vi "XYMovingPartModifying_WangYunong.vi"() -> ()   [LabVIEW 2013]
uses:
  <vilib>/Instr/_visa.llb/VISA Configure Serial Port (Instr).vi
panel:
  out "concatenated string":string
  out "read buffer":string
  out "Array 2":dbl[](array[numeric])
  out "Time2":dbl
  out "x+y":dbl
  out "Array":dbl[][](array[numeric])
  in  "stop":bool
  out "Rod Pos?":cluster{dbl[], dbl[]}(graph)
  in  "X pole":refnum<visa-resource-name>
  in  "Y pole":refnum<visa-resource-name>
  in  "Mov speed(mm/s)":dbl format="%#_13g"
  out "y resolution":dbl
  out "x resolution":dbl
  out "XY Graph":cluster{dbl[], dbl[]}(graph)
  in  "Y Center / mm":dbl format="%#_13g"
  in  "X Center / mm":dbl format="%#_13g"
  in  "Size input solution":enum16{"Dynamic Size", "Fixed Size"}(ring)=enum."Fixed Size"
  out "Time":dbl
  in  "Shape":enum16{"Self-defined", "Circle"}(ring)=enum."Circle"
  in  "Radius / mm":dbl format="%#_13g"
  in  "Precision":i32
  in  "Polygon Point":dbl[][](array[numeric])
  out "X":i32
  out "Y":i32
  out "Case":i16
  out "x-y":u32
  in  "Y move Maximum / mm":dbl
  in  "X move Maximum / mm":dbl
  in  "Y step / mm":dbl
  in  "X step / mm":dbl
  in  "Initial YPos / mm":dbl
  in  "Initial XPos / mm":dbl
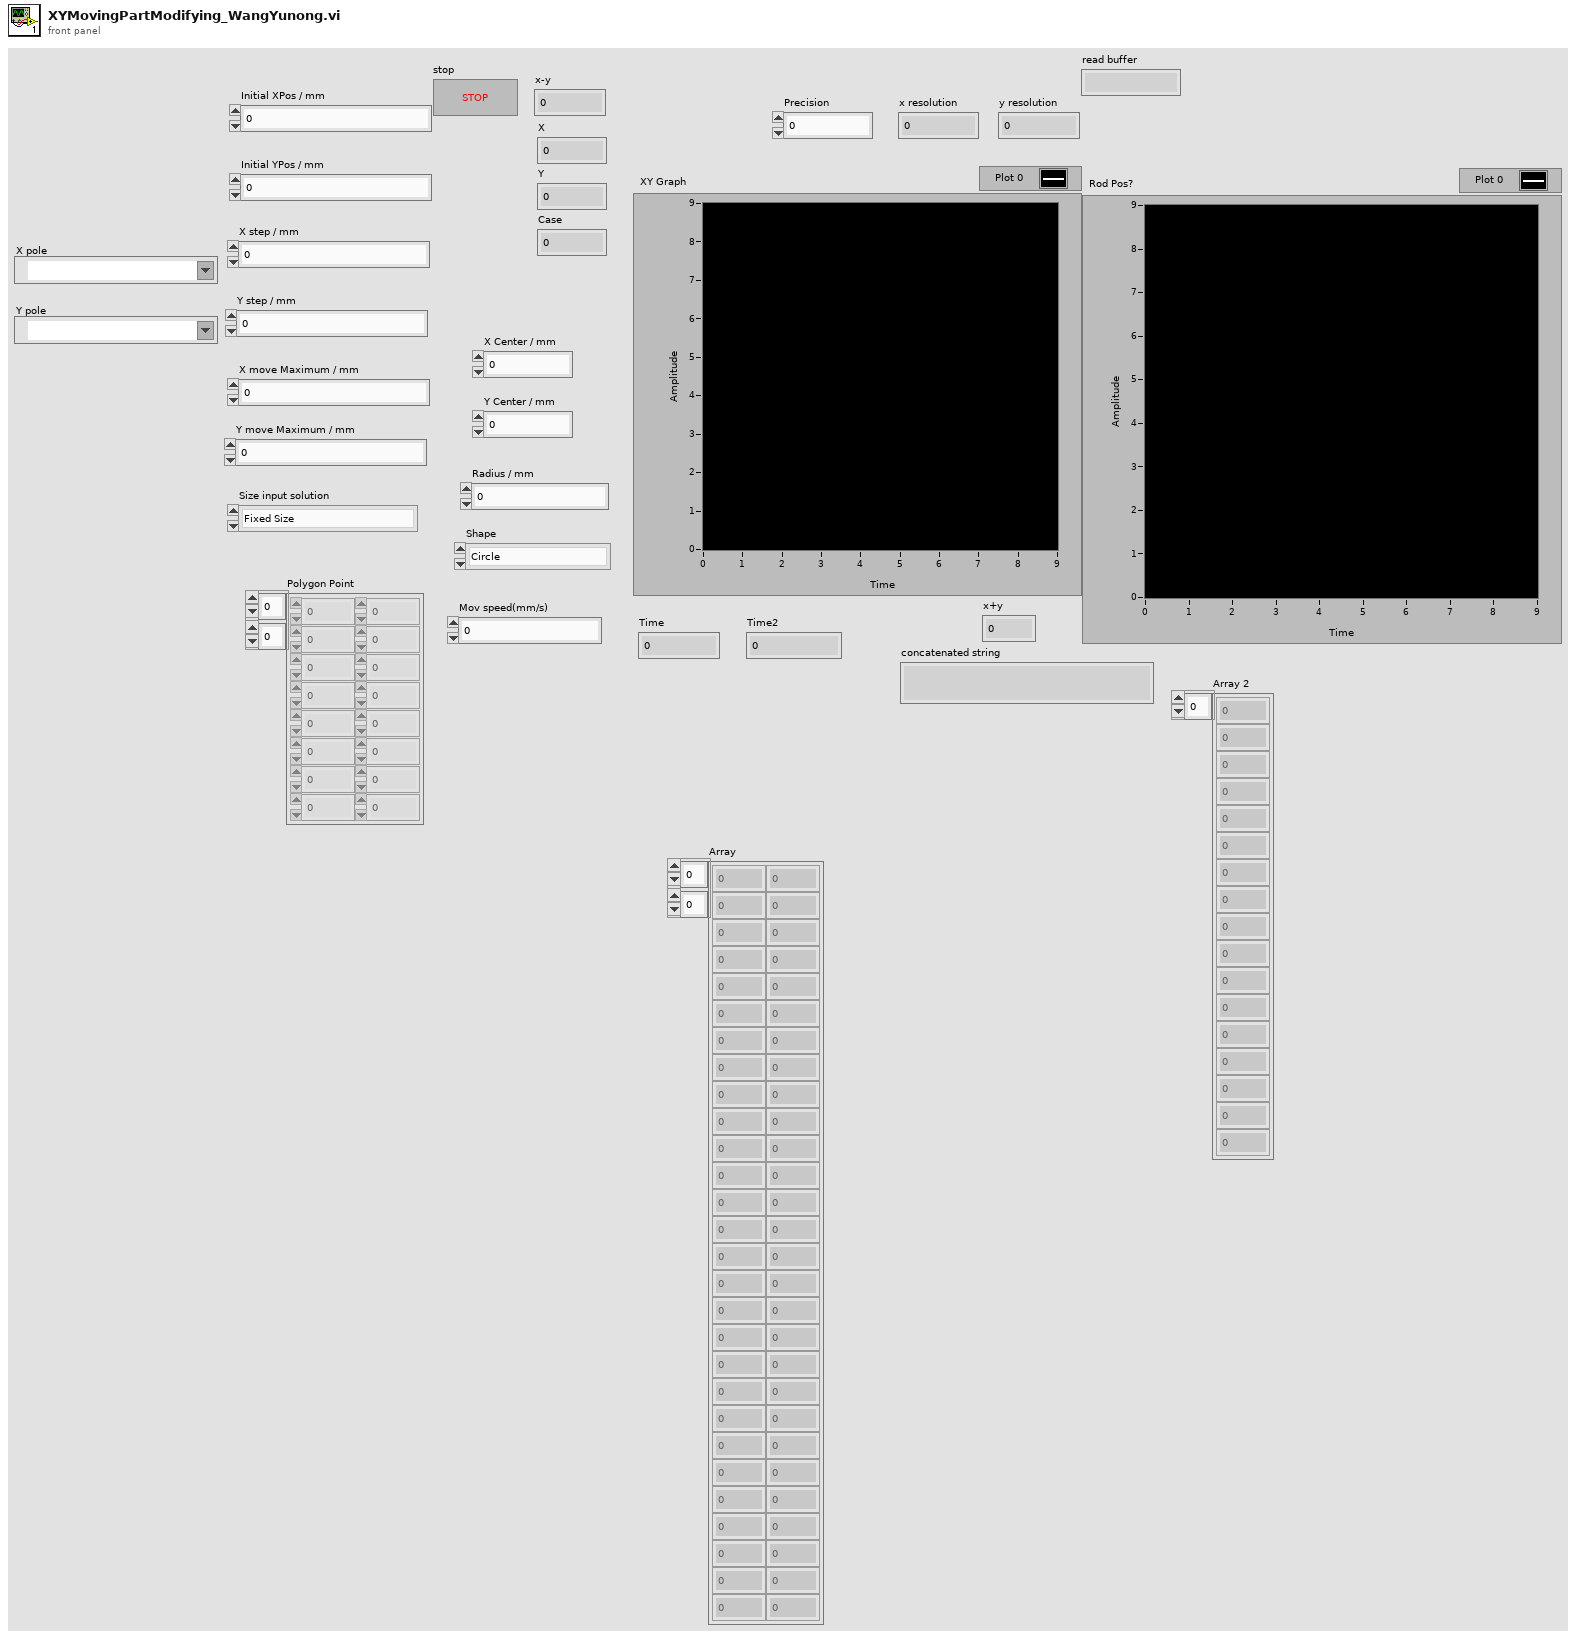
[diagram p1: front panel]
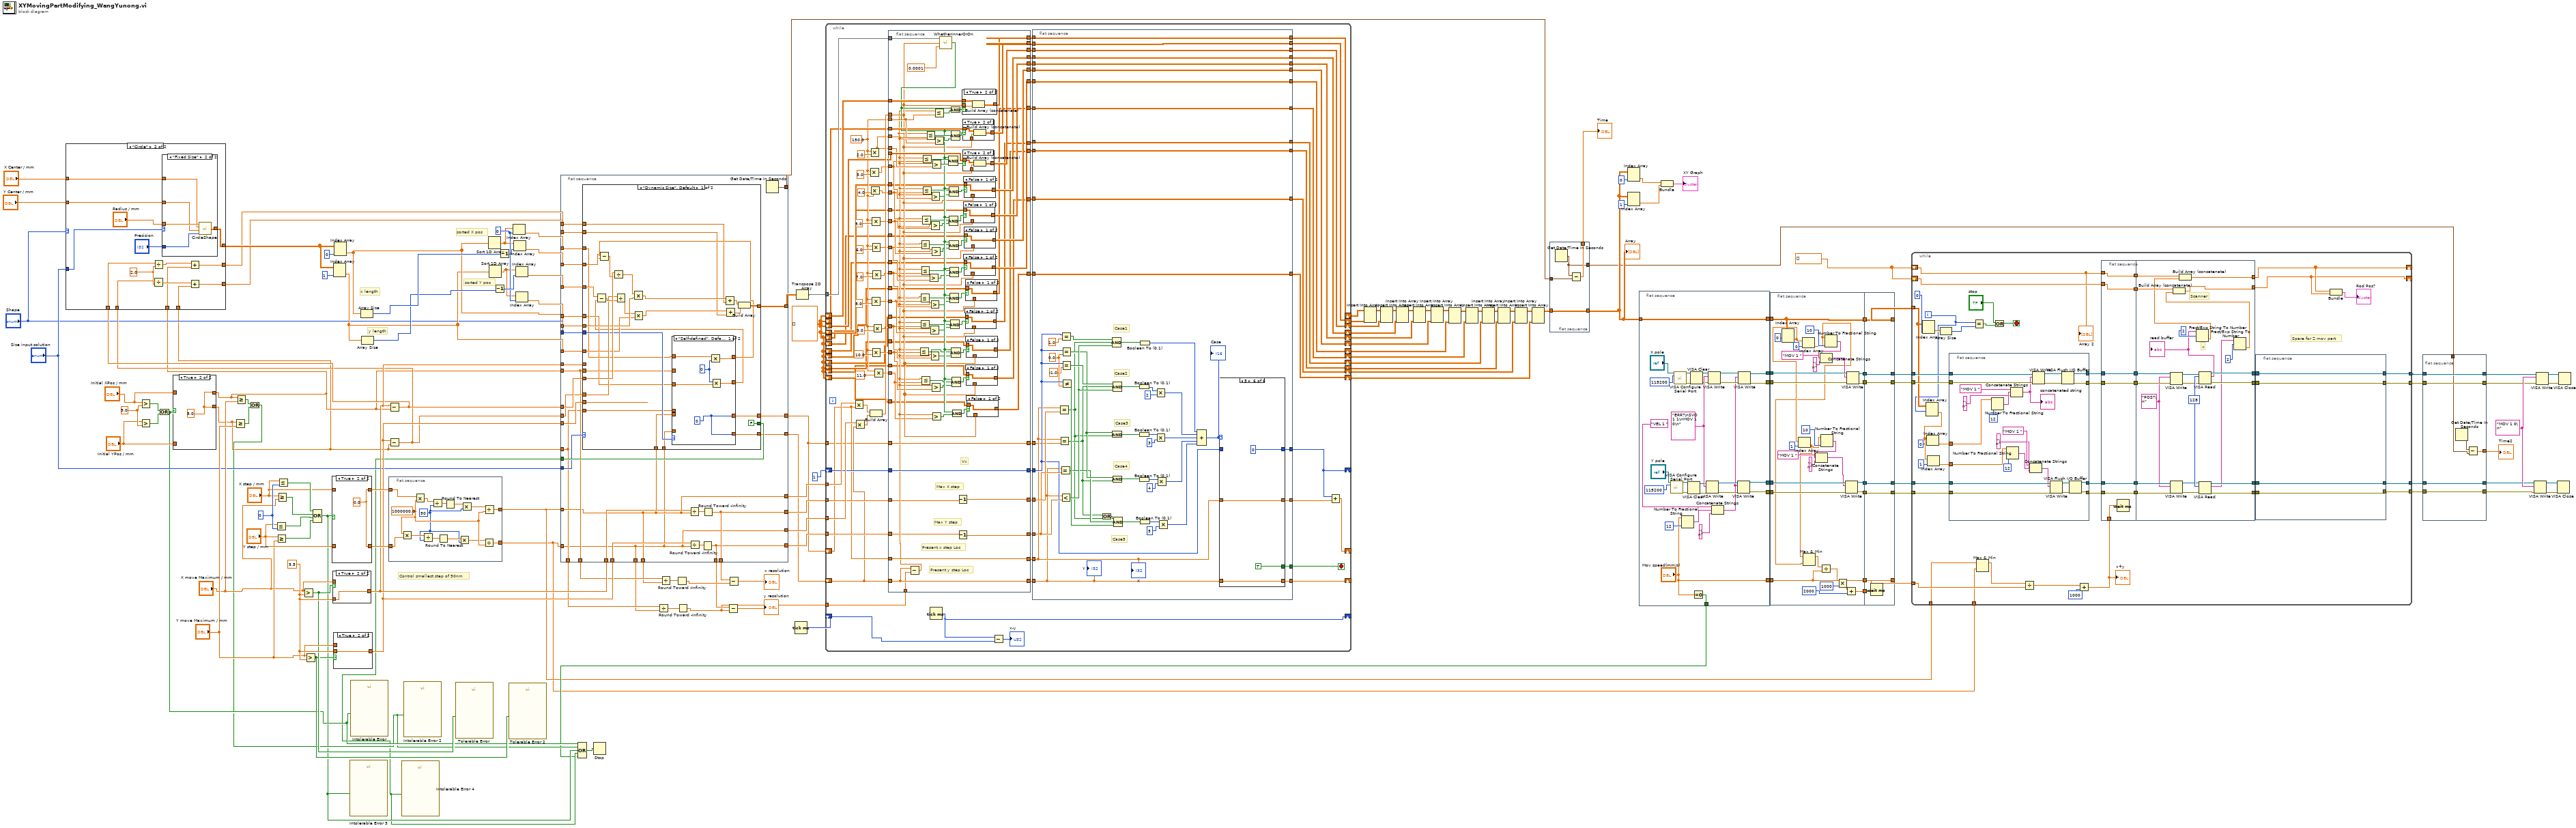
[diagram p0: block diagram]
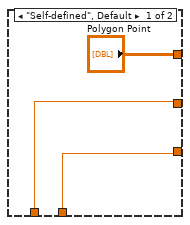
[diagram p2: hidden frame]
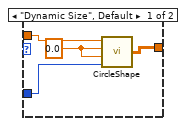
[diagram p3: hidden frame]
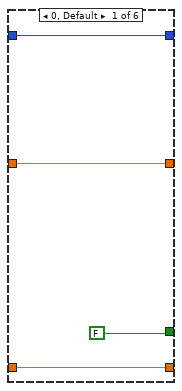
[diagram p4: hidden frame]
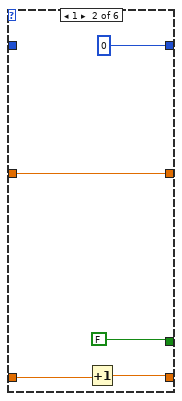
[diagram p5: hidden frame]
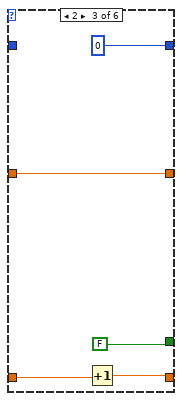
[diagram p6: hidden frame]
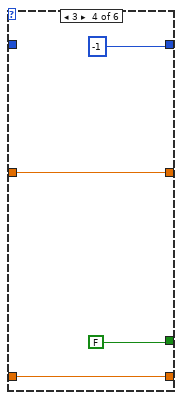
[diagram p7: hidden frame]
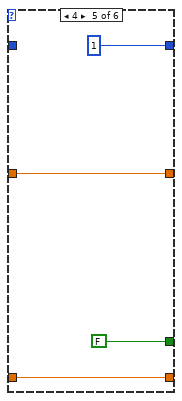
[diagram p8: hidden frame]
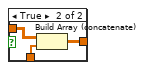
[diagram p9: hidden frame]
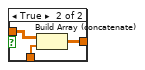
[diagram p10: hidden frame]
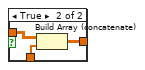
[diagram p11: hidden frame]
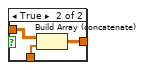
[diagram p12: hidden frame]
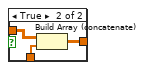
[diagram p13: hidden frame]
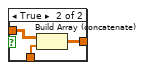
[diagram p14: hidden frame]
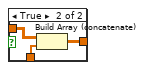
[diagram p15: hidden frame]
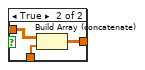
[diagram p16: hidden frame]
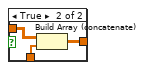
[diagram p17: hidden frame]
diagram:
  w26 = "MOV 1 0\n"
  w21 = dbl[] []
  w95 = 0 ("index")
  w61 = dbl[][] []
  w140 = 0
  w141 = 9.5
  w146 = 5.0
  # "sorted Y pos"
  # "sorted X pos"
  # "Control smallest step of 50nm"
  # "y length"
  # "x length"
  n1 = Greater?(x="Initial XPos / mm", y=w146) -> (0:w145:bool)
  n2 = Greater?(x="Initial YPos / mm", y=w146) -> (0:w144:bool)
  n3 = Or(x=w145, y=w144) -> (x .or. y?=w102:bool)
  n4 = case shown="True" w102 {
    tunnel: "Initial XPos / mm" -> [w148 _]
    tunnel: "Initial YPos / mm" -> [w147 _]
    tunnel: [w148 w149] -> w83
    tunnel: [w147 w149] -> w82
    frame False {
    }
    frame True {
      w149 = 5.0
    }
  }
  n5 = Greater Or Equal?(x=w82, y="Y move Maximum / mm") -> (x >= y?=w128:bool)
  n6 = Greater Or Equal?(x=w83, y="X move Maximum / mm") -> (x >= y?=w129:bool)
  n7 = Or(x=w129, y=w128) -> (x .or. y?=w101:bool)
  n8 = Less Or Equal?(x="Y step / mm", y=w140) -> (x <= y?=w137:bool)
  n9 = Greater Or Equal?(x="Y step / mm", y="Y move Maximum / mm") -> (x >= y?=w136:bool)
  n10 = Greater Or Equal?(x="X step / mm", y="X move Maximum / mm") -> (x >= y?=w138:bool)
  n11 = Less Or Equal?(x="X step / mm", y=w140) -> (x <= y?=w139:bool)
  n12 = Greater?(x="X move Maximum / mm", y=w141) -> (0:w127:bool)
  n13 = Greater?(x="Y move Maximum / mm", y=w141) -> (0:w126:bool)
  n14 = Compound Arithmetic op=OR(w139, w138, w137, w136) -> (w100:bool)
  n15 = case shown="True" w100 {
    tunnel: "X step / mm" -> [w151 _]
    tunnel: "Y step / mm" -> [w150 _]
    tunnel: [w151 w152] -> w125
    tunnel: [w150 w152] -> w124
    frame False {
    }
    frame True {
      w152 = 0.0
    }
  }
  n16 = case shown="True" w127 {
    tunnel: w141 -> [_ w154]
    tunnel: "X move Maximum / mm" -> [w153 _]
    tunnel: [w153 w154] -> w115
    frame False {
    }
    frame True {
    }
  }
  n17 = case shown="True" w126 {
    tunnel: w141 -> [_ w156]
    tunnel: "Y move Maximum / mm" -> [w155 _]
    tunnel: [w155 w156] -> w114
    frame False {
    }
    frame True {
    }
  }
  n18 = call "Intolerable Error 3"("Enable"=w100) -> ()  [unwired: 9 in, 2 out]
  n19 = call "Intolerable Error"("Enable"=w102) -> ()  [unwired: 9 in, 2 out]
  n20 = Subtract(x=w115, y=w83) -> (x-y=w108:dbl)
  n21 = Subtract(x=w114, y=w82) -> (x-y=w107:dbl)
  n22 = case shown="\"Circle\"" "Shape" {
    tunnel: ["Polygon Point" w172] -> w117
    tunnel: "Size input solution" -> [_ w171]
    tunnel: w108 -> [_ w167]
    tunnel: w107 -> [_ w166]
    tunnel: w82 -> [w157 w165]
    tunnel: w83 -> [w158 w164]
    tunnel: [w158 w163] -> w106
    tunnel: [w157 w162] -> w105
    tunnel: "X Center / mm" -> [_ w161]
    tunnel: "Y Center / mm" -> [_ w160]
    frame "Self-defined", Default {
    }
    frame "Circle" {
      w170 = 2.0
      n23 = Divide(x=w166, y=w170) -> (x/y=w168:dbl)
      n24 = Divide(x=w167, y=w170) -> (x/y=w169:dbl)
      n25 = case shown="\"Fixed Size\"" w171 {
        tunnel: "Radius / mm" -> [w177 w183]
        tunnel: "Precision" -> [w176 w182]
        tunnel: [w178 w181] -> w172
        tunnel: w161 -> [_ w180]
        tunnel: w160 -> [_ w179]
        frame "Dynamic Size", Default {
          w175 = 0.0 ("X initial")
          n26 = call "CircleShape.vi"("Precision"=w176, "Y initial"=w175, "X initial"=w175, "Radius"=w177) -> ("Output Point"=w178:dbl[][])
        }
        frame "Fixed Size" {
          n27 = call "CircleShape.vi"("Precision"=w182, "Y initial"=w179, "X initial"=w180, "Radius"=w183) -> ("Output Point"=w181:dbl[][])
        }
      }
      n28 = Add(x=w169, y=w164) -> (x+y=w163:dbl)
      n29 = Add(x=w168, y=w165) -> (x+y=w162:dbl)
    }
  }
  n30 = Index Array(array=w117, index (col)=1 ("disabled index (col)")) -> (element=w85:dbl[])  [unwired: 1 in]
  n31 = Index Array(array=w117, index (col)=0 ("disabled index (col)")) -> (element=w86:dbl[])  [unwired: 1 in]
  n32 = Array Size(array=w86) -> (size(s)=w88:i32)
  n33 = Array Size(array=w85) -> (size(s)=w87:i32)
  n34 = flat-sequence {
    tunnel: w125 -> [w197]
    tunnel: w124 -> [w194]
    tunnel: [w190] -> w20
    tunnel: [w189] -> w19
    frame #0 {
      w186 = 50
      w191 = 1000000.0
      n35 = Multiply(x=w191, y=w194) -> (x*y=w193:dbl)
      n36 = Multiply(x=w197, y=w191) -> (x*y=w196:dbl)
      n37 = Divide(x=w193, y=w186) -> (x/y=w192:dbl)
      n38 = Divide(x=w196, y=w186) -> (x/y=w195:dbl)
      n39 = Round To Nearest(number=w192) -> (nearest integer value=w187:dbl)
      n40 = Round To Nearest(number=w195) -> (nearest integer value=w188:dbl)
      n41 = Multiply(x=w187, y=w186) -> (x*y=w185:dbl)
      n42 = Multiply(x=w188, y=w186) -> (x*y=w184:dbl)
      n43 = Divide(x=w185, y=w191) -> (x/y=w189:dbl)
      n44 = Divide(x=w184, y=w191) -> (x/y=w190:dbl)
    }
  }
  n45 = call "Intolerable Error 4"("Enable"=w99) -> ()  [unwired: 9 in, 2 out]
  n46 = call "Intolerable Error 2"("Enable"=w101) -> ()  [unwired: 9 in, 2 out]
  n47 = call "Tolerable Error"("Enable"=w127) -> ()  [unwired: 9 in, 2 out]
  n48 = Sort 1D Array(array=w86) -> (sorted array=w93:dbl[])
  n49 = Sort 1D Array(array=w85) -> (sorted array=w94:dbl[])
  n50 = Decrement(x=w87) -> (x-1=w96:i32)
  n51 = Decrement(x=w88) -> (x-1=w97:i32)
  n52 = call "Tolerable Error 2"("Enable"=w126) -> ()  [unwired: 9 in, 2 out]
  n53 = Index Array(array=w93, index=w95) -> (element=w92:dbl)
  n54 = Index Array(array=w93, index=w97) -> (element=w91:dbl)
  n55 = Index Array(array=w94, index=w96) -> (element=w90:dbl)
  n56 = Index Array(array=w94, index=w95) -> (element=w89:dbl)
  n57 = flat-sequence {
    tunnel: w108 -> [w220]
    tunnel: w107 -> [w219]
    tunnel: w115 -> [w226]
    tunnel: w83 -> [w203]
    tunnel: w114 -> [w225]
    tunnel: w82 -> [w199]
    tunnel: [w224] -> w99
    tunnel: w20 -> [w202]
    tunnel: w19 -> [w198]
    tunnel: [w223] -> w119
    tunnel: [w201] -> w123
    tunnel: [w200] -> w122
    tunnel: [w198] -> w121
    tunnel: [w202] -> w120
    tunnel: [w218] -> w116
    tunnel: w106 -> [w217]
    tunnel: w105 -> [w216]
    tunnel: w115 -> [w215]
    tunnel: w114 -> [w214]
    tunnel: [w213] -> w110
    tunnel: [w212] -> w111
    tunnel: "Size input solution" -> [w211]
    tunnel: w92 -> [w210]
    tunnel: w91 -> [w209]
    tunnel: w90 -> [w208]
    tunnel: w89 -> [w207]
    tunnel: w86 -> [w206]
    tunnel: w85 -> [w205]
    tunnel: "Shape" -> [w204]
    tunnel: [w203] -> w72
    tunnel: [w202] -> w71
    tunnel: [w201] -> w69
    tunnel: [w200] -> w65
    tunnel: [w199] -> w64
    tunnel: [w198] -> w63
    frame #0 {
      n58 = case shown="\"Dynamic Size\", Default" w211 {
        tunnel: w206 -> [w249 w277]
        tunnel: w205 -> [w248 w276]
        tunnel: w209 -> [w255 w292]
        tunnel: w210 -> [w234 w290]
        tunnel: w208 -> [w254 w288]
        tunnel: w207 -> [w232 w285]
        tunnel: w220 -> [w253 _]
        tunnel: w219 -> [w250 _]
        tunnel: [w235 w278] -> w223
        tunnel: w226 -> [_ w291]
        tunnel: w203 -> [w243 w289]
        tunnel: w225 -> [_ w287]
        tunnel: w199 -> [w242 w286]
        tunnel: [FALSE w279] -> w224
        tunnel: w217 -> [w227 _]
        tunnel: w216 -> [w228 _]
        tunnel: w202 -> [w241 _]
        tunnel: w198 -> [w240 _]
        tunnel: [w238 w275] -> w213
        tunnel: [w239 w275] -> w212
        tunnel: w204 -> [w244 _]
        frame "Dynamic Size", Default {
          n59 = case shown="\"Self-defined\", Default" w244 {
            tunnel: w243 -> [_ w272]
            tunnel: w242 -> [_ w271]
            tunnel: w241 -> [_ w270]
            tunnel: w240 -> [_ w269]
            tunnel: [w261 w268] -> w239
            tunnel: [w261 w267] -> w238
            tunnel: w234 -> [w260 w266]
            tunnel: [w257 w265] -> w233
            tunnel: w232 -> [w259 w264]
            tunnel: [w256 w262] -> w231
            frame "Self-defined", Default {
              w258 = 0
              w261 = 0
              n60 = Multiply(x=w260, y=w258) -> (x*y=w257:dbl)
              n61 = Multiply(x=w258, y=w259) -> (x*y=w256:dbl)
            }
            frame "Circle" {
              w263 = 1.0
              n62 = Divide(x=w271, y=w269) -> (x/y=w273:dbl)
              n63 = Divide(x=w272, y=w270) -> (x/y=w274:dbl)
              n64 = Multiply(x=w266, y=w263) -> (x*y=w265:dbl)
              n65 = Multiply(x=w263, y=w264) -> (x*y=w262:dbl)
              n66 = Round Toward -Infinity(1:w274) -> (0:w268:dbl)
              n67 = Round Toward -Infinity(1:w273) -> (0:w267:dbl)
            }
          }
          n68 = Subtract(x=w254, y=w231) -> (x-y=w251:dbl)
          n69 = Subtract(x=w255, y=w233) -> (x-y=w252:dbl)
          n70 = Divide(x=w253, y=w252) -> (x/y=w230:dbl)
          n71 = Divide(x=w250, y=w251) -> (x/y=w229:dbl)
          n72 = Multiply(x=w230, y=w249) -> (x*y=w246:dbl[])
          n73 = Multiply(x=w229, y=w248) -> (x*y=w245:dbl[])
          n74 = Add(x=w246, y=w227) -> (x+y=w237:dbl[])
          n75 = Add(x=w245, y=w228) -> (x+y=w236:dbl[])
          n76 = Build Array(w237, w236) -> (w235:dbl[][])
        }
        frame "Fixed Size" {
          w275 = 0
          n77 = Greater?(x=w292, y=w291) -> (0:w283:bool)
          n78 = Less?(x=w290, y=w289) -> (x < y?=w284:bool)
          n79 = Greater?(x=w288, y=w287) -> (0:w282:bool)
          n80 = Less?(x=w285, y=w286) -> (x < y?=w281:bool)
          n81 = Compound Arithmetic op=OR(w284, w283, w282, w281) -> (w280:bool)
          n82 = case shown="True" w280 {
            tunnel: [FALSE TRUE] -> w279
            frame False {
            }
            frame True {
            }
          }
          n83 = Build Array(w277, w276) -> (w278:dbl[][])
        }
      }
      n84 = Divide(x=w215, y=w202) -> (x/y=w222:dbl)
      n85 = Divide(x=w214, y=w198) -> (x/y=w221:dbl)
      n86 = Round Toward -Infinity(1:w221) -> (0:w200:dbl)
      n87 = Round Toward -Infinity(1:w222) -> (0:w201:dbl)
      n88 = Get Date/Time In Seconds() -> (seconds since 1Jan1904=w218:timestamp)
    }
  }
  n89 = Compound Arithmetic op=OR(w102, w101, w100, w99, w27) -> (w98:bool)
  n90 = Stop(stop? (T)=w98) -> ()
  n91 = Divide(x=w64, y=w63) -> (x/y=w66:dbl)
  n92 = Divide(x=w72, y=w71) -> (x/y=w73:dbl)
  n93 = Round Toward -Infinity(1:w73) -> (0:w68:dbl)
  n94 = Round Toward -Infinity(1:w66) -> (0:w62:dbl)
  n95 = Subtract(x=w65, y=w62) -> (x-y=→"y resolution":dbl)
  n96 = Subtract(x=w69, y=w68) -> (x-y=→"x resolution":dbl)
  n97 = Tick Count (ms)() -> (millisecond timer value=w81:u32)
  n98 = Transpose 2D Array(2D array=w119) -> (transposed array=w118:dbl[][])
  n99 = while {
    tunnel: w123 -> [w367]
    tunnel: w122 -> [w365]
    tunnel: w118 -> [w373]
    tunnel: w121 -> [w377]
    tunnel: w120 -> [w378]
    shift-right: [w358] -> _
    shift-left: 1 -> [w369]
    shift-right: [w357] -> _
    shift-left: w111 -> [w363]
    shift-right: [w356] -> _
    shift-left: w110 -> [w361]
    shift-right: [w355] -> w75
    shift-left: w61 -> [w372]
    tunnel: w111 -> [w353]
    shift-right: [w351] -> _
    shift-left: w81 -> [w352]
    shift-right: [w347] -> w74
    shift-left: w61 -> [w346]
    tunnel: w62 -> [w345]
    shift-right: [w340] -> w55
    shift-left: w61 -> [w342]
    shift-right: [w319] -> w54
    shift-left: w61 -> [w321]
    shift-right: [w316] -> w53
    shift-left: w61 -> [w318]
    shift-right: [w313] -> w52
    shift-left: w61 -> [w315]
    shift-right: [w310] -> w51
    shift-left: w61 -> [w312]
    shift-right: [w307] -> w49
    shift-left: w61 -> [w309]
    shift-right: [w304] -> w47
    shift-left: w61 -> [w306]
    shift-right: [w301] -> w46
    shift-left: w61 -> [w303]
    shift-right: [w298] -> w44
    shift-left: w61 -> [w300]
    shift-right: [w295] -> w41
    shift-left: w61 -> [w297]
    stop <- w360 stop-if-true
    w329 = 150.0
    n100 = Multiply(x=w378, y=w363) -> (x*y=w376:dbl)
    n101 = Multiply(x=w377, y=w361) -> (x*y=w375:dbl)
    n102 = Multiply(x=w329, y=3.0) -> (x*y=w339:dbl)
    n103 = Multiply(x=w329, y=2.0) -> (x*y=w344:dbl)
    n104 = Multiply(x=w329, y=4.0) -> (x*y=w335:dbl)
    n105 = Multiply(x=w329, y=5.0) -> (x*y=w328:dbl)
    n106 = Multiply(x=w329, y=8.0) -> (x*y=w325:dbl)
    n107 = Multiply(x=w329, y=6.0) -> (x*y=w327:dbl)
    n108 = Multiply(x=w329, y=10.0) -> (x*y=w323:dbl)
    n109 = Build Array(w376, w375) -> (w374:dbl[])
    n110 = Multiply(x=w329, y=7.0) -> (x*y=w326:dbl)
    n111 = Multiply(x=w329, y=9.0) -> (x*y=w324:dbl)
    n112 = Multiply(x=w329, y=11.0) -> (x*y=w322:dbl)
    n113 = flat-sequence {
      tunnel: w374 -> [w491]
      tunnel: w373 -> [w538]
      tunnel: w372 -> [w528]
      tunnel: [w541] -> w371
      tunnel: [w540] -> w370
      tunnel: w369 -> [w540]
      tunnel: [w460] -> w368
      tunnel: w367 -> [w461]
      tunnel: [w458] -> w366
      tunnel: w365 -> [w459]
      tunnel: [w539] -> w364
      tunnel: w363 -> [w539]
      tunnel: [w525] -> w362
      tunnel: w361 -> [w525]
      tunnel: [w536] -> w354
      tunnel: w353 -> [w536]
      tunnel: w329 -> [w529]
      tunnel: w344 -> [w530]
      tunnel: [w527] -> w348
      tunnel: w346 -> [w526]
      tunnel: w345 -> [w524]
      tunnel: w344 -> [w518]
      tunnel: w342 -> [w520]
      tunnel: [w519] -> w341
      tunnel: w339 -> [w490]
      tunnel: w335 -> [w488]
      tunnel: w328 -> [w487]
      tunnel: w327 -> [w486]
      tunnel: w326 -> [w485]
      tunnel: w325 -> [w484]
      tunnel: w324 -> [w483]
      tunnel: w323 -> [w482]
      tunnel: w322 -> [w480]
      tunnel: w321 -> [w479]
      tunnel: [w478] -> w320
      tunnel: w318 -> [w477]
      tunnel: [w476] -> w317
      tunnel: w315 -> [w475]
      tunnel: [w474] -> w314
      tunnel: w312 -> [w473]
      tunnel: [w472] -> w311
      tunnel: w309 -> [w471]
      tunnel: [w470] -> w308
      tunnel: w306 -> [w469]
      tunnel: [w468] -> w305
      tunnel: w303 -> [w467]
      tunnel: [w466] -> w302
      tunnel: w300 -> [w465]
      tunnel: [w464] -> w299
      tunnel: w297 -> [w463]
      tunnel: [w462] -> w296
      frame #0 {
        # "Max X step"
        # "Max Y step"
        # "Present y step Loc"
        # "Present x step Loc"
        # "Vx"
        n114 = Subtract(x=w525, y=w524) -> (x-y=w481:dbl)
        n115 = Less Or Equal?(x=w481, y=w482) -> (x <= y?=w495:bool)
        n116 = Less Or Equal?(x=w481, y=w484) -> (x <= y?=w499:bool)
        n117 = Less Or Equal?(x=w481, y=w483) -> (x <= y?=w497:bool)
        n118 = Less Or Equal?(x=w481, y=w486) -> (x <= y?=w503:bool)
        n119 = Less Or Equal?(x=w481, y=w485) -> (x <= y?=w501:bool)
        n120 = Less Or Equal?(x=w481, y=w480) -> (x <= y?=w493:bool)
        n121 = Less Or Equal?(x=w481, y=w487) -> (x <= y?=w505:bool)
        n122 = Less Or Equal?(x=w481, y=w490) -> (x <= y?=w522:bool)
        n123 = Less Or Equal?(x=w481, y=w488) -> (x <= y?=w507:bool)
        n124 = Less Or Equal?(x=w481, y=w530) -> (x <= y?=w532:bool)
        n125 = Greater?(x=w481, y=w486) -> (0:w500:bool)
        n126 = Greater?(x=w481, y=w484) -> (0:w496:bool)
        n127 = Greater?(x=w481, y=w485) -> (0:w498:bool)
        n128 = Greater?(x=w481, y=w483) -> (0:w494:bool)
        n129 = Greater?(x=w481, y=w488) -> (0:w504:bool)
        n130 = Greater?(x=w481, y=w490) -> (0:w506:bool)
        n131 = Greater?(x=w481, y=w487) -> (0:w502:bool)
        n132 = Greater?(x=w481, y=w482) -> (0:w492:bool)
        n133 = Greater?(x=w481, y=w518) -> (0:w521:bool)
        n134 = Greater?(x=w481, y=w480) -> (0:w489:bool)
        n135 = Less Or Equal?(x=w481, y=w529) -> (x <= y?=w534:bool)
        n136 = Greater?(x=w481, y=w529) -> (0:w531:bool)
        n137 = call "WhetherInnerOrOn.vi"("Error permitted"=0.0001, "JudgePoint"=w491, "InputPolygon"=w538) -> ("Point on or inside?"=w508:bool)
        n138 = Compound Arithmetic op=AND(w508, w522, w521) -> (w523:bool)
        n139 = Compound Arithmetic op=AND(w508, w505, w504) -> (w516:bool)
        n140 = And(x=w508, y=w534) -> (x .and. y?=w535:bool)
        n141 = Compound Arithmetic op=AND(w508, w507, w506) -> (w517:bool)
        n142 = Compound Arithmetic op=AND(w508, w503, w502) -> (w515:bool)
        n143 = Compound Arithmetic op=AND(w508, w501, w500) -> (w514:bool)
        n144 = Compound Arithmetic op=AND(w508, w499, w498) -> (w513:bool)
        n145 = Compound Arithmetic op=AND(w508, w497, w496) -> (w512:bool)
        n146 = Compound Arithmetic op=AND(w508, w532, w531) -> (w533:bool)
        n147 = Compound Arithmetic op=AND(w508, w495, w494) -> (w511:bool)
        n148 = Compound Arithmetic op=AND(w508, w493, w492) -> (w510:bool)
        n149 = Compound Arithmetic op=AND(w508, w489) -> (w509:bool)
        n150 = Decrement(x=w461) -> (x-1=w460:dbl)
        n151 = Decrement(x=w459) -> (x-1=w458:dbl)
        n152 = case shown="True" w535 {
          tunnel: w528 -> [w586 w589]
          tunnel: w491 -> [_ w588]
          tunnel: [w586 w587] -> w541
          frame False {
          }
          frame True {
            n153 = Build Array (concatenate)(w589, w588) -> (w587:dbl[][])
          }
        }
        n154 = case shown="True" w533 {
          tunnel: w491 -> [_ w585]
          tunnel: w526 -> [w582 w584]
          tunnel: [w582 w583] -> w527
          frame False {
          }
          frame True {
            n155 = Build Array (concatenate)(w584, w585) -> (w583:dbl[][])
          }
        }
        n156 = case shown="True" w523 {
          tunnel: w491 -> [_ w581]
          tunnel: w520 -> [w578 w580]
          tunnel: [w578 w579] -> w519
          frame False {
          }
          frame True {
            n157 = Build Array (concatenate)(w580, w581) -> (w579:dbl[][])
          }
        }
        n158 = case shown="False" w516 {
          tunnel: w491 -> [_ w545]
          tunnel: [w542 w544] -> w476
          tunnel: w477 -> [w542 w543]
          frame False {
          }
          frame True {
            n159 = Build Array (concatenate)(w543, w545) -> (w544:dbl[][])
          }
        }
        n160 = case shown="False" w517 {
          tunnel: w491 -> [_ w577]
          tunnel: [w574 w576] -> w478
          tunnel: w479 -> [w574 w575]
          frame False {
          }
          frame True {
            n161 = Build Array (concatenate)(w575, w577) -> (w576:dbl[][])
          }
        }
        n162 = case shown="False" w514 {
          tunnel: w491 -> [_ w569]
          tunnel: [w566 w568] -> w472
          tunnel: w473 -> [w566 w567]
          frame False {
          }
          frame True {
            n163 = Build Array (concatenate)(w567, w569) -> (w568:dbl[][])
          }
        }
        n164 = case shown="False" w515 {
          tunnel: w491 -> [_ w573]
          tunnel: [w570 w572] -> w474
          tunnel: w475 -> [w570 w571]
          frame False {
          }
          frame True {
            n165 = Build Array (concatenate)(w571, w573) -> (w572:dbl[][])
          }
        }
        n166 = case shown="False" w512 {
          tunnel: w491 -> [_ w561]
          tunnel: [w558 w560] -> w468
          tunnel: w469 -> [w558 w559]
          frame False {
          }
          frame True {
            n167 = Build Array (concatenate)(w559, w561) -> (w560:dbl[][])
          }
        }
        n168 = case shown="False" w513 {
          tunnel: w491 -> [_ w565]
          tunnel: [w562 w564] -> w470
          tunnel: w471 -> [w562 w563]
          frame False {
          }
          frame True {
            n169 = Build Array (concatenate)(w563, w565) -> (w564:dbl[][])
          }
        }
        n170 = case shown="False" w511 {
          tunnel: w491 -> [_ w557]
          tunnel: [w554 w556] -> w466
          tunnel: w467 -> [w554 w555]
          frame False {
          }
          frame True {
            n171 = Build Array (concatenate)(w555, w557) -> (w556:dbl[][])
          }
        }
        n172 = case shown="False" w510 {
          tunnel: w491 -> [_ w553]
          tunnel: [w550 w552] -> w464
          tunnel: w465 -> [w550 w551]
          frame False {
          }
          frame True {
            n173 = Build Array (concatenate)(w551, w553) -> (w552:dbl[][])
          }
        }
        n174 = case shown="False" w509 {
          tunnel: w491 -> [_ w549]
          tunnel: [w546 w548] -> w462
          tunnel: w463 -> [w546 w547]
          frame False {
          }
          frame True {
            n175 = Build Array (concatenate)(w547, w549) -> (w548:dbl[][])
          }
        }
      }
    }
    n176 = Tick Count (ms)() -> (millisecond timer value=w351:u32)
    n177 = Subtract(x=w351, y=w352) -> (x-y=→"x-y":u32)
    n178 = flat-sequence {
      tunnel: w371 -> [w394]
      tunnel: w370 -> [w401]
      tunnel: w368 -> [w431]
      tunnel: w366 -> [w429]
      tunnel: w364 -> [w400]
      tunnel: w362 -> [w399]
      tunnel: [w398] -> w360
      tunnel: [w397] -> w359
      tunnel: [w396] -> w358
      tunnel: [w395] -> w356
      tunnel: [w394] -> w355
      tunnel: w354 -> [w393]
      tunnel: w348 -> [w389]
      tunnel: [w389] -> w347
      tunnel: w341 -> [w388]
      tunnel: [w388] -> w340
      tunnel: [w387] -> w319
      tunnel: w320 -> [w387]
      tunnel: w317 -> [w386]
      tunnel: [w386] -> w316
      tunnel: w314 -> [w385]
      tunnel: [w385] -> w313
      tunnel: w311 -> [w384]
      tunnel: [w384] -> w310
      tunnel: w308 -> [w383]
      tunnel: [w383] -> w307
      tunnel: w305 -> [w382]
      tunnel: [w382] -> w304
      tunnel: w302 -> [w381]
      tunnel: [w381] -> w301
      tunnel: w299 -> [w380]
      tunnel: [w380] -> w298
      tunnel: w296 -> [w379]
      tunnel: [w379] -> w295
      frame #0 {
        w391 = 0.0
        # "Case5"
        # "Case4"
        # "Case3"
        # "Case2"
        # "Case1"
        n179 = Equal?(x=w400, y=w431) -> (x = y?=w421:bool)
        n180 = Equal?(x=w400, y=w393) -> (x = y?=w422:bool)
        n181 = Equal?(x=w399, y=w429) -> (x = y?=w423:bool)
        n182 = Less?(x=w399, y=w429) -> (x < y?=w427:bool)
        n183 = Equal?(x=w401, y=1.0) -> (x = y?=w430:bool)
        n184 = Equal?(x=w401, y=w391) -> (x = y?=w426:bool)
        n185 = Equal?(x=w401, y=-1.0) -> (x = y?=w428:bool)
        n186 = Not Equal?(x=w401, y=w391) -> (x != y?=w424:bool)
        n187 = Or(x=w422, y=w421) -> (x .or. y?=w425:bool)
        n188 = Compound Arithmetic op=AND(w430, w421, w427) -> (w420:bool)
        n189 = Compound Arithmetic op=AND(w426, w421) -> (w418:bool)
        n190 = Compound Arithmetic op=AND(w428, w422, w427) -> (w419:bool)
        n191 = Compound Arithmetic op=AND(w426, w422) -> (w417:bool)
        n192 = Compound Arithmetic op=AND(w425, w423, w424) -> (w416:bool)
        n193 = Boolean To (0,1)(Boolean=w418) -> (0, 1=w411:i16)
        n194 = Boolean To (0,1)(Boolean=w417) -> (0, 1=w409:i16)
        n195 = Boolean To (0,1)(Boolean=w419) -> (0, 1=w413:i16)
        n196 = Boolean To (0,1)(Boolean=w420) -> (0, 1=w414:i16)
        n197 = Boolean To (0,1)(Boolean=w416) -> (0, 1=w407:i16)
        n198 = Multiply(x=w413, y=i16 2) -> (x*y=w405:i16)
        n199 = Multiply(x=w411, y=i16 3) -> (x*y=w404:i16)
        n200 = Multiply(x=w409, y=i16 4) -> (x*y=w403:i16)
        n201 = Multiply(x=w407, y=i16 5) -> (x*y=w402:i16)
        n202 = Compound Arithmetic op=ADD(w414, w405, w404, w403, w402) -> (w415:i16)
        "Case" <- w415
        n203 = case shown="5" w415 {
          tunnel: w401 -> [w435 _ _ _ _ _]
          tunnel: w400 -> [w434 w437 w442 w448 w452 w457]
          tunnel: w399 -> [w433 w439 w444 w447 w451 w456]
          tunnel: [w435 0 0 -1 1 0] -> w396
          tunnel: [w434 w437 w442 w448 w452 w457] -> w397
          tunnel: [w433 w438 w443 w447 w451 w456] -> w395
          tunnel: [FALSE FALSE FALSE FALSE FALSE TRUE] -> w398
          frame 0, Default {
          }
          frame 1 {
            n204 = Increment(x=w439) -> (x+1=w438:dbl)
          }
          frame 2 {
            n205 = Increment(x=w444) -> (x+1=w443:dbl)
          }
          frame 3 {
          }
          frame 4 {
          }
          frame 5 {
          }
        }
        "X" <- w400
        "Y" <- w399
      }
    }
    n206 = Add(x=w358, y=w359) -> (x+y=w357:dbl)
  }
  n207 = Insert Into Array(array=w75, new element=w74) -> (w60:dbl[][])  [unwired: 2 in]
  n208 = Insert Into Array(array=w60, new element=w55) -> (w59:dbl[][])  [unwired: 2 in]
  n209 = Insert Into Array(array=w59, new element=w54) -> (w58:dbl[][])  [unwired: 2 in]
  n210 = Insert Into Array(array=w58, new element=w53) -> (w57:dbl[][])  [unwired: 2 in]
  n211 = Insert Into Array(array=w57, new element=w52) -> (w56:dbl[][])  [unwired: 2 in]
  n212 = Insert Into Array(array=w56, new element=w51) -> (w50:dbl[][])  [unwired: 2 in]
  n213 = Insert Into Array(array=w50, new element=w49) -> (w48:dbl[][])  [unwired: 2 in]
  n214 = Insert Into Array(array=w48, new element=w47) -> (w45:dbl[][])  [unwired: 2 in]
  n215 = Insert Into Array(array=w45, new element=w46) -> (w43:dbl[][])  [unwired: 2 in]
  n216 = Insert Into Array(array=w43, new element=w44) -> (w42:dbl[][])  [unwired: 2 in]
  n217 = Insert Into Array(array=w42, new element=w41) -> (w40:dbl[][])  [unwired: 2 in]
  n218 = flat-sequence {
    tunnel: [w593] -> w18
    tunnel: w40 -> [w593]
    tunnel: w116 -> [w592]
    tunnel: [w591] -> w112
    tunnel: [w590] -> w9
    frame #0 {
      n219 = Get Date/Time In Seconds() -> (seconds since 1Jan1904=w590:timestamp)
      n220 = Subtract(x=w590, y=w592) -> (x-y=w591:dbl)
    }
  }
  n221 = Index Array(array=w18, index (col)=0 ("disabled index (col)")) -> (element=w78:dbl[])  [unwired: 1 in]
  n222 = Index Array(array=w18, index (col)=1 ("disabled index (col)")) -> (element=w79:dbl[])  [unwired: 1 in]
  n223 = flat-sequence {
    tunnel: [w617] -> w39
    tunnel: w18 -> [w617]
    tunnel: [w610] -> w38
    tunnel: [w609] -> w37
    tunnel: [w614] -> w36
    tunnel: [w613] -> w35
    tunnel: [w603] -> w27
    tunnel: ["Mov speed(mm/s)"] -> w29
    frame #0 {
      w618 = "ERR?\nSVO 1 1\nMOV 1 0\n"
      n224 = call-poly "VISA Configure Serial Port"("VISA resource name"="Y pole", "baud rate (9600)"=u32 115200) -> ("VISA resource name out"=w597:refnum<visa-resource-name>, "error out"=w596:errorcluster)  [unwired: 12 in]
      n225 = call-poly "VISA Configure Serial Port"("VISA resource name"="X pole", "baud rate (9600)"=u32 115200) -> ("VISA resource name out"=w600:refnum<visa-resource-name>, "error out"=w601:errorcluster)  [unwired: 12 in]
      n226 = Number To Fractional String(number="Mov speed(mm/s)", precision (6)=i16 12) -> (F-format string=w607:string)  [unwired: 2 in]
      n227 = VISA Clear(VISA resource name=w597, error in (no error)=w596) -> (VISA resource name out=w595:refnum<visa-resource-name>, error out=w594:errorcluster)
      n228 = VISA Clear(VISA resource name=w600, error in (no error)=w601) -> (VISA resource name out=w599:refnum<visa-resource-name>, error out=w598:errorcluster)
      n229 = Equal To 0?(x="Mov speed(mm/s)") -> (x = 0?=w603:bool)
      n230 = VISA Write(VISA resource name=w595, write buffer=w618, error in (no error)=w594) -> (VISA resource name out=w616:refnum<visa-resource-name>, error out=w615:errorcluster)  [unwired: 1 out]
      n231 = VISA Write(VISA resource name=w599, write buffer=w618, error in (no error)=w598) -> (VISA resource name out=w612:refnum<visa-resource-name>, error out=w611:errorcluster)  [unwired: 1 out]
      n232 = Concatenate Strings("VEL 1 ", w607, "\n") -> (w604:string)
      n233 = VISA Write(VISA resource name=w616, write buffer=w604, error in (no error)=w615) -> (VISA resource name out=w614:refnum<visa-resource-name>, error out=w613:errorcluster)  [unwired: 1 out]
      n234 = VISA Write(VISA resource name=w612, write buffer=w604, error in (no error)=w611) -> (VISA resource name out=w610:refnum<visa-resource-name>, error out=w609:errorcluster)  [unwired: 1 out]
    }
  }
  n235 = Bundle(w78, w79) -> (→"XY Graph":cluster{dbl[], dbl[]})  [unwired: 1 in]
  n236 = flat-sequence {
    tunnel: w39 -> [w646]
    tunnel: w38 -> [w654]
    tunnel: w37 -> [w652]
    tunnel: w36 -> [w650]
    tunnel: w35 -> [w648]
    tunnel: w29 -> [w627]
    tunnel: [w646] -> w7
    tunnel: [w653] -> w6
    tunnel: [w651] -> w5
    tunnel: [w649] -> w4
    tunnel: [w647] -> w3
    tunnel: [w627] -> w2
    tunnel: [w626] -> w1
    tunnel: [w656] -> w28
    tunnel: [w657] -> w30
    tunnel: [w658] -> w31
    tunnel: [w659] -> w32
    tunnel: [w660] -> w33
    tunnel: [w661] -> w34
    tunnel: w7 -> [w661]
    tunnel: w6 -> [w660]
    tunnel: w5 -> [w659]
    tunnel: w4 -> [w658]
    tunnel: w3 -> [w657]
    tunnel: w2 -> [w656]
    tunnel: w1 -> [w655]
    frame #0 {
      n237 = Index Array(array=w646, index (row)=0) -> (element=w632:dbl[])  [unwired: 1 in]
      n238 = Index Array(array=w632, index=1) -> (element=w631:dbl)
      n239 = Index Array(array=w632, index=0) -> (element=w630:dbl)
      n240 = Max & Min(x=w631, y=w630) -> (max(x,y)=w628:dbl)  [unwired: 1 out]
      n241 = Divide(x=w628, y=w627) -> (x/y=w623:dbl)
      n242 = Number To Fractional String(number=w631, precision (6)=i16 10) -> (F-format string=w638:string)  [unwired: 2 in]
      n243 = Concatenate Strings("MOV 1 ", w638, "\n" ("string")) -> (w635:string)
      n244 = Number To Fractional String(number=w630, precision (6)=i16 10) -> (F-format string=w643:string)  [unwired: 2 in]
      n245 = Concatenate Strings("MOV 1 ", w643, "\n" ("string")) -> (w640:string)
      n246 = Multiply(x=w623, y=1000) -> (x*y=w625:dbl)
      n247 = VISA Write(VISA resource name=w650, write buffer=w635, error in (no error)=w648) -> (VISA resource name out=w649:refnum<visa-resource-name>, error out=w647:errorcluster)  [unwired: 1 out]
      n248 = Add(x=w625, y=u32 2000 ("milliseconds to wait")) -> (x+y=w626:dbl)
      n249 = VISA Write(VISA resource name=w654, write buffer=w640, error in (no error)=w652) -> (VISA resource name out=w653:refnum<visa-resource-name>, error out=w651:errorcluster)  [unwired: 1 out]
    }
    frame #1 {
      n250 = Wait (ms)(milliseconds to wait=w655) -> ()  [unwired: 1 out]
    }
  }
  n251 = while {
    tunnel: w34 -> [w702]
    tunnel: w33 -> [w706]
    tunnel: w32 -> [w705]
    tunnel: w31 -> [w704]
    tunnel: w30 -> [w703]
    shift-right: [w666] -> _
    shift-left: w21 -> [w663]
    tunnel: w28 -> [w691]
    tunnel: [w688] -> w16
    tunnel: [w686] -> w14
    tunnel: [w684] -> w12
    tunnel: [w683] -> w10
    shift-right: [w665] -> _
    shift-left: w21 -> [w668]
    tunnel: w20 -> [w672]
    tunnel: w19 -> [w673]
    i -> [w662]
    stop <- w676 stop-if-true
    # "Spare for Z mov part"
    n252 = Index Array(array=w702, index (col)=0 ("disabled index (col)")) -> (element=w707:dbl[])  [unwired: 1 in]
    n253 = Index Array(array=w702, index (row)=w662) -> (element=w695:dbl[])  [unwired: 1 in]
    n254 = Index Array(array=w695, index=0) -> (element=w693:dbl)
    n255 = Index Array(array=w695, index=1) -> (element=w692:dbl)
    n256 = Array Size(array=w707) -> (size(s)=w670:i32)
    n257 = flat-sequence {
      tunnel: w706 -> [w767]
      tunnel: w705 -> [w766]
      tunnel: w704 -> [w755]
      tunnel: w703 -> [w754]
      tunnel: [w749] -> w701
      tunnel: [w748] -> w700
      tunnel: [w745] -> w698
      tunnel: [w744] -> w699
      tunnel: w693 -> [w760]
      tunnel: w692 -> [w752]
      frame #0 {
        n258 = Number To Fractional String(number=w760, precision (6)=i16 12) -> (F-format string=w763:string)  [unwired: 2 in]
        n259 = Number To Fractional String(number=w752, precision (6)=i16 12) -> (F-format string=w758:string)  [unwired: 2 in]
        n260 = Concatenate Strings("MOV 1 ", w763, "\n") -> (w765:string)
        "concatenated string" <- w765
        n261 = Concatenate Strings("MOV 1 ", w758, "\n" ("string")) -> (w753:string)
        n262 = VISA Write(VISA resource name=w767, write buffer=w765, error in (no error)=w766) -> (VISA resource name out=w751:refnum<visa-resource-name>, error out=w750:errorcluster)  [unwired: 1 out]
        n263 = VISA Write(VISA resource name=w755, write buffer=w753, error in (no error)=w754) -> (VISA resource name out=w747:refnum<visa-resource-name>, error out=w746:errorcluster)  [unwired: 1 out]
        n264 = VISA Flush I/O Buffer(VISA resource name=w751, error in (no error)=w750) -> (VISA resource name out=w749:refnum<visa-resource-name>, error out=w748:errorcluster)  [unwired: 1 in]
        n265 = VISA Flush I/O Buffer(VISA resource name=w747, error in (no error)=w746) -> (VISA resource name out=w745:refnum<visa-resource-name>, error out=w744:errorcluster)  [unwired: 1 in]
      }
    }
    n266 = Equal?(x=w662, y=w670) -> (x = y?=w675:bool)
    n267 = Max & Min(x=w672, y=w673) -> (max(x,y)=w671:dbl)  [unwired: 1 out]
    n268 = Or(x="stop", y=w675) -> (x .or. y?=w676:bool)
    n269 = Divide(x=w671, y=w691) -> (x/y=w690:dbl)
    n270 = Add(x=w690, y=1000) -> (x+y=w677:dbl)
    "x+y" <- w677
    n271 = flat-sequence {
      tunnel: w701 -> [w719]
      tunnel: w700 -> [w718]
      tunnel: w699 -> [w716]
      tunnel: w698 -> [w717]
      tunnel: [w719] -> w681
      tunnel: [w718] -> w680
      tunnel: [w717] -> w679
      tunnel: [w716] -> w678
      tunnel: w677 -> [w715]
      tunnel: w663 -> [w714]
      tunnel: [w714] -> w669
      tunnel: w668 -> [w713]
      tunnel: [w713] -> w667
      tunnel: [w740] -> w682
      tunnel: [w741] -> w685
      tunnel: [w742] -> w687
      tunnel: [w743] -> w689
      tunnel: w681 -> [w738]
      tunnel: w680 -> [w736]
      tunnel: w679 -> [w734]
      tunnel: w678 -> [w732]
      tunnel: w669 -> [w725]
      tunnel: w667 -> [w724]
      tunnel: [w723] -> w666
      tunnel: [w722] -> w665
      frame #0 {
        n272 = Wait (ms)(milliseconds to wait=w715) -> ()  [unwired: 1 out]
      }
      frame #1 {
        w730 = "POS?\n"
        w739 = u32 128 ("byte count")
        # "Scanner"
        # "x"
        n273 = VISA Write(VISA resource name=w738, write buffer=w730, error in (no error)=w736) -> (VISA resource name out=w737:refnum<visa-resource-name>, error out=w735:errorcluster)  [unwired: 1 out]
        n274 = VISA Write(VISA resource name=w734, write buffer=w730, error in (no error)=w732) -> (VISA resource name out=w733:refnum<visa-resource-name>, error out=w731:errorcluster)  [unwired: 1 out]
        n275 = VISA Read(VISA resource name=w737, byte count=w739, error in (no error)=w735) -> (VISA resource name out=w743:refnum<visa-resource-name>, read buffer=w727:string, error out=w742:errorcluster)  [unwired: 1 out]
        "read buffer" <- w727
        n276 = Fract/Exp String To Number(string=w727, offset=2) -> (number=w721:dbl)  [unwired: 2 in, 1 out]
        n277 = Build Array (concatenate)(w725, w721) -> (w723:dbl[])
        n278 = VISA Read(VISA resource name=w733, byte count=w739, error in (no error)=w731) -> (VISA resource name out=w741:refnum<visa-resource-name>, read buffer=w726:string, error out=w740:errorcluster)  [unwired: 1 out]
        n279 = Fract/Exp String To Number(string=w726, offset=2) -> (number=w720:dbl)  [unwired: 2 in, 1 out]
        n280 = Build Array (concatenate)(w724, w720) -> (w722:dbl[])
      }
    }
    n281 = flat-sequence {
      tunnel: w689 -> [w712]
      tunnel: [w712] -> w688
      tunnel: [w711] -> w686
      tunnel: w687 -> [w711]
      tunnel: [w710] -> w684
      tunnel: w685 -> [w710]
      tunnel: [w709] -> w683
      tunnel: w682 -> [w709]
      frame #0 {
      }
    }
    n282 = Bundle(w666, w665) -> (→"Rod Pos?":cluster{dbl[], dbl[]})  [unwired: 1 in]
    "Array 2" <- w663
  }
  n283 = flat-sequence {
    tunnel: [w774] -> w17
    tunnel: w16 -> [w774]
    tunnel: [w773] -> w15
    tunnel: w14 -> [w773]
    tunnel: [w772] -> w13
    tunnel: w12 -> [w772]
    tunnel: [w771] -> w11
    tunnel: w10 -> [w771]
    tunnel: w9 -> [w769]
    tunnel: [w768] -> w8
    frame #0 {
      n284 = Get Date/Time In Seconds() -> (seconds since 1Jan1904=w770:timestamp)
      n285 = Subtract(x=w770, y=w769) -> (x-y=w768:dbl)
    }
  }
  n286 = VISA Write(VISA resource name=w13, write buffer=w26, error in (no error)=w11) -> (VISA resource name out=w23:refnum<visa-resource-name>, error out=w22:errorcluster)  [unwired: 1 out]
  n287 = VISA Write(VISA resource name=w17, write buffer=w26, error in (no error)=w15) -> (VISA resource name out=w24:refnum<visa-resource-name>, error out=w25:errorcluster)  [unwired: 1 out]
  n288 = VISA Close(VISA resource name=w23, error in (no error)=w22) -> ()  [unwired: 1 out]
  n289 = VISA Close(VISA resource name=w24, error in (no error)=w25) -> ()  [unwired: 1 out]
  "Time" <- w112
  "Array" <- w18
  "Time2" <- w8
